vi "Has More Points.vi"(0 "eye scan point iterator":refnum<class "niHighSpeedSerial N Point Eye Scan Point Iterator v1 Host.lvclass">, 11 "error in":errorcluster) -> (4 "eye scan point iterator out":refnum<class "niHighSpeedSerial N Point Eye Scan Point Iterator v1 Host.lvclass">, 6 "has more points?":bool, 15 "error out":errorcluster)   [LabVIEW 2014, in "niHighSpeedSerial N Point Eye Scan Point Iterator v1 Host.lvclass"]
doc: "Returns true if there are more points available that have not yet been measured.\n\n<B>Input Parameters</B>\n\n<B>eye scan point iterator</B> is the incoming wire for the Eye Scan Point Iterator class object\n\n<B>error in</B> describes error conditions that occur before this node runs. This input provides standard 'error in' functionality.\n\n<B>Output Parameters</B>\n\n<B>eye scan point iterator out</B> is the outgoing wire for the Eye Scan Point Iterator class object\n\n<B>has more points?</B> is true if there are more points available that have not yet been measured.\n\n<B>error out</B> contains error information. This output provides standard 'error out' functionality."
uses:
  <instrlib>/niHighSpeedSerial/Eye Scan/v1/Host/Impl/N Pt Iter/niHighSpeedSerial N Point Eye Scan Point Iterator v1 Host.lvclass
  <instrlib>/niHighSpeedSerial/Eye Scan/v1/Host/Impl/N Pt Iter/niHighSpeedSerial N Point Eye Scan Point Iterator v1 Host.lvclass/niHighSpeedSerial N Point Eye Scan Point Iterator v1 Host.ctl
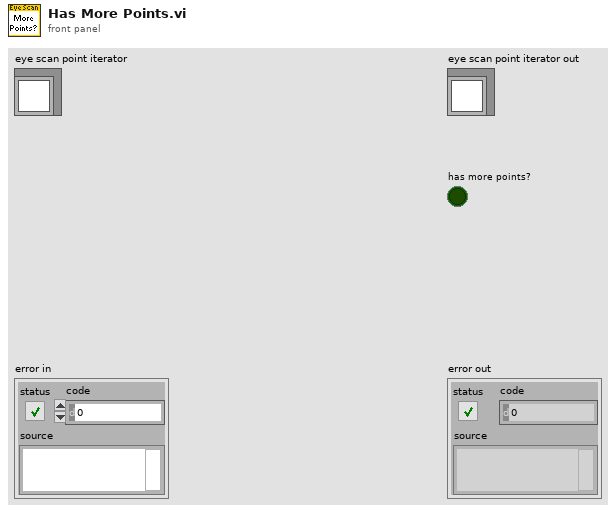
[diagram p1: front panel]
types:
  T1 = typedef "niHighSpeedSerial Eye Scan Common v1 Host.lvlib/Point.ctl" = cluster{"point offsets":T2, "sample count":u64, "error count":u64, "bit error rate":dbl}
  T2 = typedef "niHighSpeedSerial Eye Scan Common v1 Host.lvlib/Point Offsets.ctl" = cluster{"horizontal offset":i16, "vertical offset":i8}
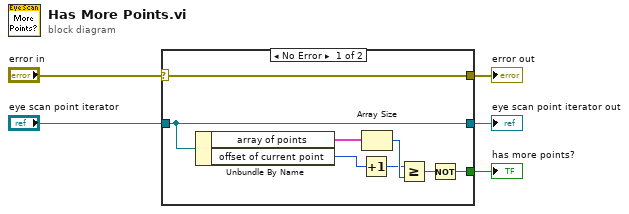
[diagram p0: block diagram]
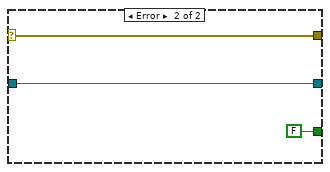
[diagram p2: hidden frame]
diagram:
  n1 = case shown="No Error" "error in" {
    selector: "error in" -> [w13 w16]
    tunnel: [w13 w16] -> w4
    tunnel: [w6 w15] -> w3
    tunnel: "eye scan point iterator" -> [w6 w15]
    tunnel: [w12 FALSE ("Has More Points?")] -> w1
    frame No Error {
      n2 = Unbundle By Name(w6) -> ("array of points"=w11:T1[], "offset of current point"=w10:i32)
      n3 = Increment(x=w10) -> (x+1=w7:i32)
      n4 = Array Size(array=w11) -> (size(s)=w9:i32)
      n5 = Greater Or Equal?(x=w7, y=w9) -> (x >= y?=w8:bool)
      n6 = Not(x=w8) -> (.not. x?=w12:bool)
    }
    frame Error {
    }
  }
  "error out" <- w4
  "eye scan point iterator out" <- w3
  "has more points?" <- w1
